vi "DeleteService.vi"(8 "error in (no error)":errorcluster, 11 "service name":string) -> (0 "error out":errorcluster)   [LabVIEW 2021]
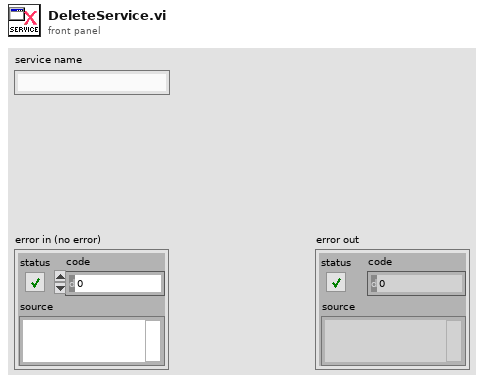
[diagram p1: front panel]
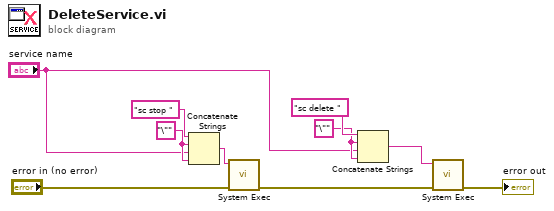
[diagram p0: block diagram]
diagram:
  w2 = "\"" ("string")
  w3 = "\"" ("string")
  n1 = Concatenate Strings("sc stop " ("string"), w3, "service name", w3) -> (w5:string)
  n2 = call <vilib>:"System Exec.vi"("error in (no error)"="error in (no error)", "command line"=w5) -> ("error out"=w6:errorcluster)  [unwired: 6 in, 3 out]
  n3 = Concatenate Strings("sc delete " ("string"), w2, "service name", w2) -> (w8:string)
  n4 = call <vilib>:"System Exec.vi"("error in (no error)"=w6, "command line"=w8) -> ("error out"=→"error out":errorcluster)  [unwired: 6 in, 3 out]
